vi "eec 6700 Perform Test in Program Mode.vi"() -> ()   [LabVIEW 2014]
doc: "Configures the instrument to Program mode and starts the test.\nThe instrument has 50 memory locations with 9 steps for each memory location.\n\nPress stop button to end the test process.\n\nNote :1. In Firmware version 2.0, the Voltage Limits and Frequency limits are removed from program mode. Its possible to configure the limits in version 1.06 only.\n\n2. Also the Output angle (Start and End) Angle is used as a step parameter in firmware version 2 and system parameter in the firmware version 1.06 respectively.\n\n3. In firmware version 1.06, Enable Surge-Drop Mode is a system parameter (common for all steps and memory. Change in mode affect all steps and memory)\n\n4. In the firmware version 2.0 and above ,surge drop can be used only in the Program Mode and it is a step parameter."
uses:
  <instrlib>/eec 6700/eec 6700.lvlib
panel:
  in  "Timeout (10000 ms)":u32=10000
  in  "Starting Step (1)":i32=1
  in  "Enable Over Current Fold Back (F:Disable)":bool
  in  "Start Angle (0)":i32 min=0 max=359
  in  "End Angle: (0)":i32 min=0 max=359
  in  "Frequency High Limit (500 Hz)":dbl=500.0 min=0.0 max=500.0 format="%.1f"
  in  "Frequency Low Limit (40 Hz)":dbl=40.0 min=0.0 max=500.0 format="%.1f"
  in  "Voltage Low Limit (0 V)":dbl min=0.0 max=400.0 format="%.1f"
  in  "Voltage High Limit (300 V)":dbl=300.0 min=0.0 max=400.0 format="%.1f"
  out "Status Byte Register Cluster":T1={"All Pass"=TRUE, "Fail"=FALSE, "Abort"=FALSE, "Test in Process"=FALSE, "Message Available"=FALSE, "Event Summary Bit"=FALSE, "Not Used"=FALSE, "Prompt"=FALSE}
  in  "Stop":bool
  in  "VISA resource name":refnum<visa-resource-name>="COM1"
  out "Test Meter Data Output":T2={"Memory"=1.0, "Step"=4.0, "Timer (s)"=1.0, "Frequency (Hz)"=60.0, "Voltage (V)"=125.0, "RMS Current (A)"=0.0, "Peak Current (A)"=0.0, "Power (W)"=0.0, "Power Factor"=0.0, "Status"="Pass"} {"Frequency (Hz)" format="%.1f"; "Voltage (V)" format="%.1f"; "RMS Current (A)" format="%.3f"; "Power (W)" format="%.1f"; "Peak Current (A)" format="%.1f"; "Power Factor" format="%.3f"; "Timer (s)" format="%.1f"}
  in  "Memory Cycle (1)":i32=1 min=0 max=9999 step=1
  in  "Memory (1)":i32=1 min=1 max=50 step=1
  in  "Single Step Mode (F:Disable)":bool
  in  "Loop Cycle (1)":i32=1 min=0 max=9999 step=1
  in  "Step Parameters":T3(array[cluster])=[{"Current High Limit (0 A)"=0.0, "Current Peak High Limit (0 A)"=0.0, "Output AC Voltage (115 V) "=115.0, "Enable Step Connection (F:Disable)"=TRUE, "Step (1)"=1, "Step Cycle (1)"=1, "Power Low Limit (0 W)"=0.0, "Power High Limit (0 W)"=0.0, "Power Factor Low Limit (0)"=0.0, "Power Factor High Limit (0)"=0.0, "Current Low Limit (0 A)"=0.0, "Current Peak Low Limit (0 A)"=0.0, "Dwell (1 s)"=3.0, "Ramp Down Time (0 s)"=2.0, "Delay (0.5 s)"=1.0, "Ramp Up Time (0 s)"=2.0, "Surge Drop Duration (0 ms)"=0.0, "Surge Drop Voltage (100 V) "=100.0, "Surge Drop Start Time (0 ms)"=0.0, "Enable  Continuous Surge Drop (F:Disable)"=FALSE, "Output AC Voltage Frequency (60  Hz)"=60.0, "Voltage Range Mode (1:Auto)"=1, "Enable Surge Drop (F:Disable) "=FALSE, "Step Prompt"={"Enable Prompt"=FALSE, "Prompt ( )"=""}}, {"Current High Limit (0 A)"=0.0, "Current Peak High Limit (0 A)"=8.1387e-320, "Output AC Voltage (115 V) "=110.0, "Enable Step Connection (F:Disable)"=TRUE, "Step (1)"=2, "Step Cycle (1)"=1, "Power Low Limit (0 W)"=0.0, "Power High Limit (0 W)"=0.0, "Power Factor Low Limit (0)"=1.35542481148e-312, "Power Factor High Limit (0)"=0.0, "Current Low Limit (0 A)"=0.0, "Current Peak Low Limit (0 A)"=0.0, "Dwell (1 s)"=15.0, "Ramp Down Time (0 s)"=1.0, "Delay (0.5 s)"=0.5, "Ramp Up Time (0 s)"=1.0, "Surge Drop Duration (0 ms)"=0.0, "Surge Drop Voltage (100 V) "=100.0, "Surge Drop Start Time (0 ms)"=0.0, "Enable  Continuous Surge Drop (F:Disable)"=FALSE, "Output AC Voltage Frequency (60  Hz)"=60.0, "Voltage Range Mode (1:Auto)"=1, "Enable Surge Drop (F:Disable) "=FALSE, "Step Prompt"={"Enable Prompt"=FALSE, "Prompt ( )"=""}}, {"Current High Limit (0 A)"=0.0, "Current Peak High Limit (0 A)"=0.0, "Output AC Voltage (115 V) "=120.0, "Enable Step Connection (F:Disable)"=TRUE, "Step (1)"=3, "Step Cycle (1)"=1, "Power Low Limit (0 W)"=0.0, "Power High Limit (0 W)"=0.0, "Power Factor Low Limit (0)"=0.0, "Power Factor High Limit (0)"=0.0, "Current Low Limit (0 A)"=0.0, "Current Peak Low Limit (0 A)"=0.0, "Dwell (1 s)"=1.0, "Ramp Down Time (0 s)"=0.0, "Delay (0.5 s)"=0.5, "Ramp Up Time (0 s)"=0.0, "Surge Drop Duration (0 ms)"=0.0, "Surge Drop Voltage (100 V) "=100.0, "Surge Drop Start Time (0 ms)"=0.0, "Enable  Continuous Surge Drop (F:Disable)"=FALSE, "Output AC Voltage Frequency (60  Hz)"=65.0, "Voltage Range Mode (1:Auto)"=1, "Enable Surge Drop (F:Disable) "=FALSE, "Step Prompt"={"Enable Prompt"=FALSE, "Prompt ( )"=""}}, {"Current High Limit (0 A)"=0.0, "Current Peak High Limit (0 A)"=0.0, "Output AC Voltage (115 V) "=125.0, "Enable Step Connection (F:Disable)"=FALSE, "Step (1)"=4, "Step Cycle (1)"=1, "Power Low Limit (0 W)"=0.0, "Power High Limit (0 W)"=0.0, "Power Factor Low Limit (0)"=0.0, "Power Factor High Limit (0)"=0.0, "Current Low Limit (0 A)"=0.0, "Current Peak Low Limit (0 A)"=0.0, "Dwell (1 s)"=1.0, "Ramp Down Time (0 s)"=0.0, "Delay (0.5 s)"=0.5, "Ramp Up Time (0 s)"=0.0, "Surge Drop Duration (0 ms)"=0.0, "Surge Drop Voltage (100 V) "=100.0, "Surge Drop Start Time (0 ms)"=0.0, "Enable  Continuous Surge Drop (F:Disable)"=FALSE, "Output AC Voltage Frequency (60  Hz)"=60.0, "Voltage Range Mode (1:Auto)"=1, "Enable Surge Drop (F:Disable) "=FALSE, "Step Prompt"={"Enable Prompt"=FALSE, "Prompt ( )"=""}}] {"Voltage Range Mode (1:Auto)" items=["High", "Auto"]; "Output AC Voltage Frequency (60  Hz)" min=45.0 max=500.0 format="%.1p"; "Surge Drop Start Time (0 ms)" min=0.0 max=99.0; "Surge Drop Voltage (100 V)" min=0.0 max=300.0 format="%#.1f"; "Surge Drop Duration (0 ms)" min=0.0 max=99.0; "Ramp Up Time (0 s)" min=0.0 max=999.9 format="%.1f"; "Delay (0.5 s)" min=0.5 max=999.9 format="%.1f"; "Ramp Down Time (0 s)" min=0.0 max=999.9 format="%.1f"; "Dwell (1 s)" min=0.5 max=999.9 format="%.1f"; "Current Peak Low Limit (0 A)" min=0.0 max=152.0 format="%.3f"; "Current Low Limit (0 A)" min=0.0 max=36.8 format="%.3f"; "Power Factor High Limit (0)" min=0.0 max=1.0 format="%.3f"; "Power Factor Low Limit (0)" min=0.0 max=1.0 format="%.3f"; "Power High Limit (0 W)" min=0.0 max=4000.0 format="%.1f"; "Power Low Limit (0 W)" min=0.0 max=4000.0 format="%.1f"; "Step Cycle (1)" min=0 max=9999 step=1; "Step (1)" min=1 max=9 step=1; "Output AC Voltage (115 V)" min=0.0 max=300.0 format="%.1f"; "Current Peak High Limit (0 A)" min=0.0 max=152.0 format="%.3f"; "Current High Limit (0 A)" min=0.0 max=36.8 format="%.3f"}
  out "Error Out":errorcluster
  # "eec 6700 PROGRAM MODE - EXAMPLE"
  # "Note :\n1. Configure the Parameters (Select the instrument VISA resource, voltage etc.,)\n2. Run this VI"
  # "The Step connect mode is used to connect or disconnect one step from another.\nPlease Switch it ON to connect from Step 1 to Step 2."
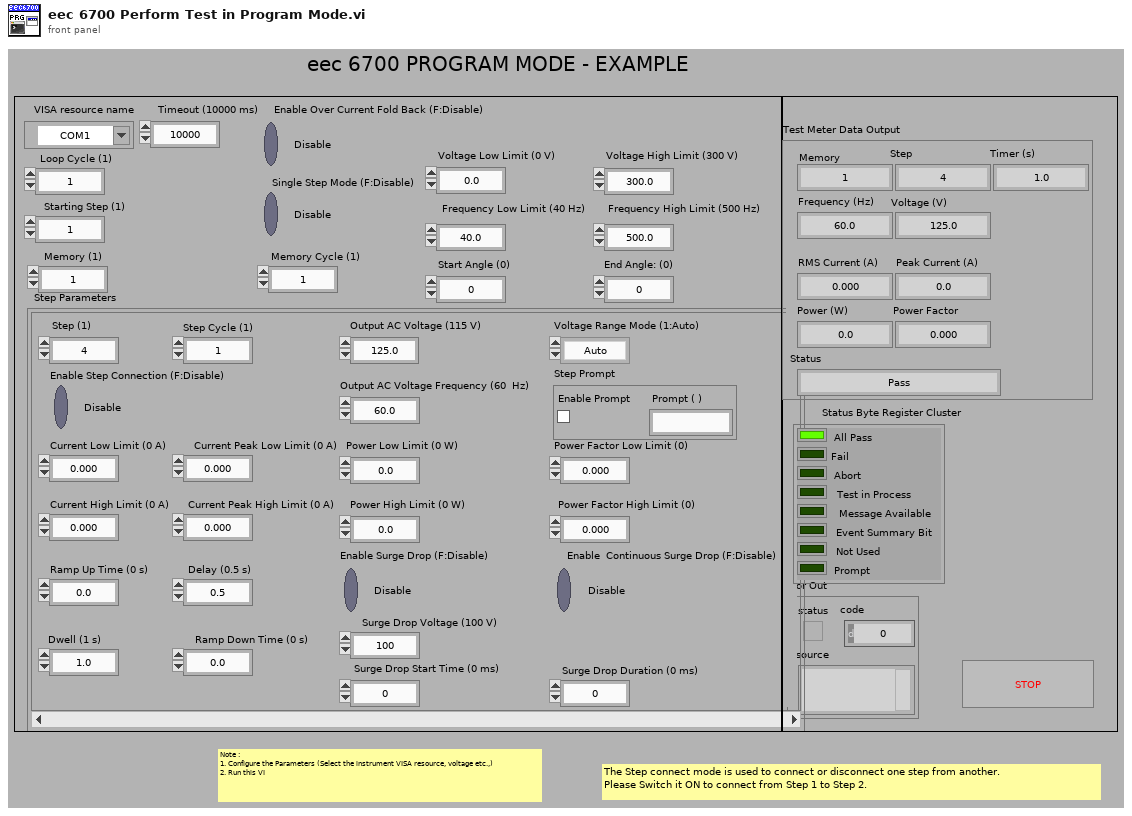
[diagram p1: front panel]
types:
  T1 = cluster{"All Pass":bool, "Fail":bool, "Abort":bool, "Test in Process":bool, "Message Available":bool, "Event Summary Bit":bool, "Not Used":bool, "Prompt":bool}
  T2 = cluster{"Memory":dbl, "Step":dbl, "Timer (s)":dbl, "Frequency (Hz)":dbl, "Voltage (V)":dbl, "RMS Current (A)":dbl, "Peak Current (A)":dbl, "Power (W)":dbl, "Power Factor":dbl, "Status":string}
  T3 = cluster{"Current High Limit (0 A)":dbl, "Current Peak High Limit (0 A)":dbl, "Output AC Voltage (115 V) ":dbl, "Enable Step Connection (F:Disable)":bool, "Step (1)":i32, "Step Cycle (1)":i32, "Power Low Limit (0 W)":dbl, "Power High Limit (0 W)":dbl, "Power Factor Low Limit (0)":dbl, "Power Factor High Limit (0)":dbl, "Current Low Limit (0 A)":dbl, "Current Peak Low Limit (0 A)":dbl, "Dwell (1 s)":dbl, "Ramp Down Time (0 s)":dbl, "Delay (0.5 s)":dbl, "Ramp Up Time (0 s)":dbl, "Surge Drop Duration (0 ms)":dbl, "Surge Drop Voltage (100 V) ":dbl, "Surge Drop Start Time (0 ms)":dbl, "Enable  Continuous Surge Drop (F:Disable)":bool, "Output AC Voltage Frequency (60  Hz)":dbl, "Voltage Range Mode (1:Auto)":u16, "Enable Surge Drop (F:Disable) ":bool, "Step Prompt":cluster{"Enable Prompt":bool, "Prompt ( )":string}}[]
  T4 = cluster{"Baud Rate":u32, "Parity":u16, "Data Bits":u16, "Stop Bits":u16, "Flow Control":u16}
  T5 = cluster{"Enable Prompt":bool, "Prompt ( )":string}
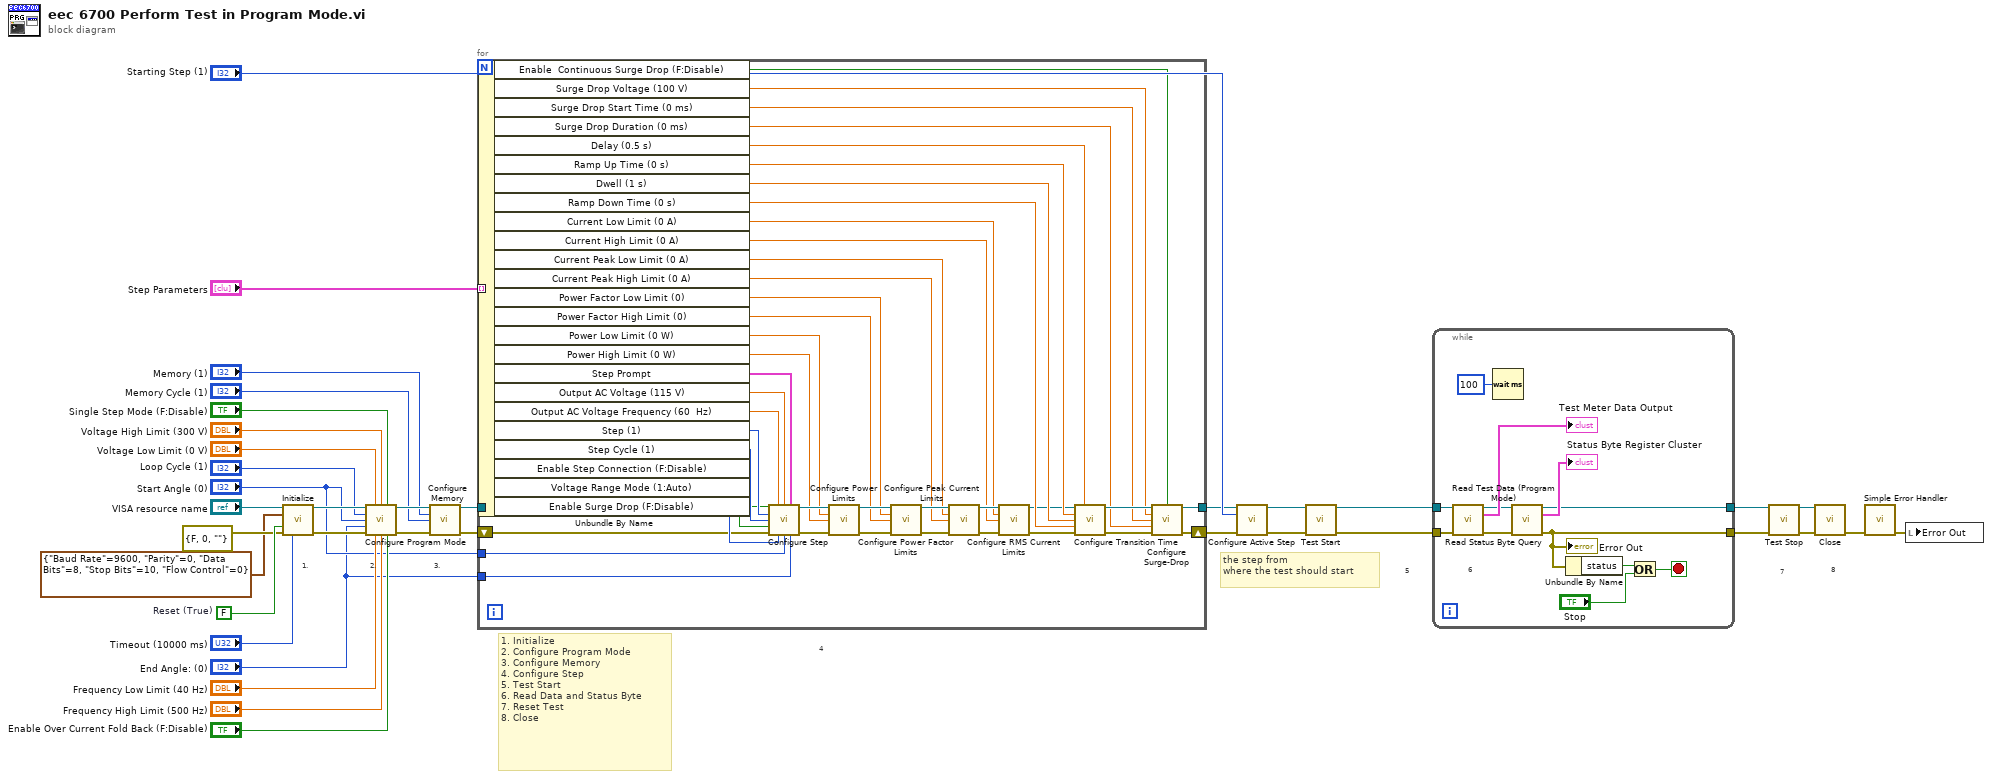
[diagram p0: block diagram]
diagram:
  w34 = FALSE  # Reset (True)
  # "the step from \nwhere the test should start"
  # "5"
  # "4"
  # "1. Initialize\n2. Configure Program Mode\n3. Configure Memory\n4. Configure Step\n5. Test Start\n6. Read Data and Status Byte\n7. Reset Test\n8. Close"
  # "7"
  # "8"
  # "1."
  # "3."
  # "2."
  n1 = call <instrlib>:"Initialize.vi"("VISA resource name"="VISA resource name", "Serial Configuration"=T4 {"Baud Rate"=9600, "Parity"=0, "Data Bits"=8, "Stop Bits"=10, "Flow Control"=0}, "Reset (True)"=w34, "error in (no error)"=errorcluster {"status"=FALSE, "code"=0, "source"=""}, "Timeout (10000 ms)"="Timeout (10000 ms)") -> ("VISA resource name out"=w33:refnum<visa-resource-name>, "error out"=w35:errorcluster)  [unwired: 9 in]
  n2 = call <instrlib>:"Configure Program Mode.vi"("VISA resource name"=w33, "Voltage Low Limit (0 V)"="Voltage Low Limit (0 V)", "Voltage High Limit (300 V)"="Voltage High Limit (300 V)", "Single Step Mode (F:Disable)"="Single Step Mode (F:Disable)", "Loop Cycle (1)"="Loop Cycle (1)", "Start Angle (0)"="Start Angle (0)", "End Angle: (0)"="End Angle: (0)", "error in (no error)"=w35, "Frequency Low Limit (40 Hz)"="Frequency Low Limit (40 Hz)", "Frequency High Limit (500 Hz)"="Frequency High Limit (500 Hz)", "Enable Over Current Fold Back (F:Disable)"="Enable Over Current Fold Back (F:Disable)") -> ("VISA resource name out"=w32:refnum<visa-resource-name>, "error out"=w31:errorcluster)  [unwired: 3 in]
  n3 = call <instrlib>:"Configure Memory.vi"("VISA resource name"=w32, "Memory (1)"="Memory (1)", "Memory Cycle (1)"="Memory Cycle (1)", "error in (no error)"=w31) -> ("VISA resource name out"=w8:refnum<visa-resource-name>, "error out"=w7:errorcluster)  [unwired: 10 in]
  n4 = for {
    tunnel: "Step Parameters" -> [w77] mode=indexing
    shift-right: [w79] -> w3
    shift-left: w7 -> [w41]
    tunnel: [w78] -> w4
    tunnel: w8 -> [w42]
    tunnel: "Start Angle (0)" -> [w40]
    tunnel: "End Angle: (0)" -> [w39]
    n5 = Unbundle By Name(w77) -> ("Enable  Continuous Surge Drop (F:Disable)"=w45:bool, "Surge Drop Voltage (100 V)"=w53:dbl, "Surge Drop Start Time (0 ms)"=w54:dbl, "Surge Drop Duration (0 ms)"=w55:dbl, "Delay (0.5 s)"=w65:dbl, "Ramp Up Time (0 s)"=w64:dbl, "Dwell (1 s)"=w59:dbl, "Ramp Down Time (0 s)"=w58:dbl, "Current Low Limit (0 A)"=w46:dbl, "Current High Limit (0 A)"=w37:dbl, "Current Peak Low Limit (0 A)"=w52:dbl, "Current Peak High Limit (0 A)"=w51:dbl, "Power Factor Low Limit (0)"=w72:dbl, "Power Factor High Limit (0)"=w71:dbl, "Power Low Limit (0 W)"=w70:dbl, "Power High Limit (0 W)"=w69:dbl, "Step Prompt"=w38:T5, "Output AC Voltage (115 V)"=w56:dbl, "Output AC Voltage Frequency (60  Hz)"=w57:dbl, "Step (1)"=w44:i32, "Step Cycle (1)"=w67:i32, "Enable Step Connection (F:Disable)"=w68:bool, "Voltage Range Mode (1:Auto)"=w66:u16, "Enable Surge Drop (F:Disable)"=w43:bool)
    n6 = call <instrlib>:"Configure Step.vi"("VISA resource name"=w42, "Output AC Voltage Frequency (60  Hz)"=w57, "Output AC Voltage (115 V)"=w56, "Step Prompt"=w38, "Step (1)"=w44, "Step Cycle (1)"=w67, "Enable Step Connection (F:Disable)"=w68, "error in (no error)"=w41, "Voltage Range Mode (1:Auto)"=w66, "Start Angle (0)"=w40, "End Angle: (0)"=w39) -> ("VISA resource name out"=w76:refnum<visa-resource-name>, "error out"=w75:errorcluster)  [unwired: 3 in]
    n7 = call <instrlib>:"Configure Power Limits.vi"("VISA resource name"=w76, "Power Low Limit (0 W)"=w70, "Power High Limit (0 W)"=w69, "error in (no error)"=w75) -> ("VISA resource name out"=w74:refnum<visa-resource-name>, "error out"=w73:errorcluster)  [unwired: 10 in]
    n8 = call <instrlib>:"Configure Power Factor Limits.vi"("VISA resource name"=w74, "Power Factor Low Limit (0)"=w72, "Power Factor High Limit (0)"=w71, "error in (no error)"=w73) -> ("VISA resource name out"=w63:refnum<visa-resource-name>, "error out"=w62:errorcluster)  [unwired: 10 in]
    n9 = call <instrlib>:"Configure Peak Current Limits.vi"("VISA resource name"=w63, "Current Peak Low Limit (0 A)"=w52, "Current Peak High Limit (0 A)"=w51, "error in (no error)"=w62) -> ("VISA resource name out"=w50:refnum<visa-resource-name>, "error out"=w49:errorcluster)  [unwired: 10 in]
    n10 = call <instrlib>:"Configure RMS Current Limits.vi"("VISA resource name"=w50, "Current Low Limit (0 A)"=w46, "Current High Limit (0 A)"=w37, "error in (no error)"=w49) -> ("VISA resource name out"=w47:refnum<visa-resource-name>, "error out"=w48:errorcluster)  [unwired: 10 in]
    n11 = call <instrlib>:"Configure Transition Time.vi"("VISA resource name"=w47, "Delay (0.5 s)"=w65, "Ramp Up Time (0 s)"=w64, "Dwell (1 s)"=w59, "Ramp Down Time (0 s)"=w58, "error in (no error)"=w48) -> ("VISA resource name out"=w60:refnum<visa-resource-name>, "error out"=w61:errorcluster)  [unwired: 8 in]
    n12 = call <instrlib>:"Configure Surge-Drop.vi"("VISA resource name"=w60, "Enable Surge Drop (F:Disable)"=w43, "Enable  Continuous Surge Drop (F:Disable)"=w45, "Surge Drop Voltage (100 V)"=w53, "Surge Drop Start Time (0 ms)"=w54, "Surge Drop Duration (0 ms)"=w55, "error in (no error)"=w61) -> ("VISA resource name out"=w78:refnum<visa-resource-name>, "error out"=w79:errorcluster)  [unwired: 7 in]
  }
  n13 = call <instrlib>:"Configure Active Step.vi"("VISA resource name"=w4, "Step (1)"="Starting Step (1)", "error in (no error)"=w3) -> ("VISA resource name out"=w16:refnum<visa-resource-name>, "error out"=w15:errorcluster)  [unwired: 11 in]
  n14 = call <instrlib>:"Test Start.vi"("VISA resource name"=w16, "error in (no error)"=w15) -> ("VISA resource name out"=w2:refnum<visa-resource-name>, "error out"=w1:errorcluster)  [unwired: 12 in]
  n15 = while {
    tunnel: [w84] -> w24
    tunnel: [w80] -> w22
    tunnel: w2 -> [w91]
    tunnel: w1 -> [w90]
    stop <- w81 stop-if-true
    # "6"
    n16 = call <instrlib>:"Read Test Data (Program Mode).vi"("VISA resource name"=w91, "error in (no error)"=w90) -> ("VISA resource name out"=w85:refnum<visa-resource-name>, "Test Meter Data Output"=→"Test Meter Data Output":T2, "error out"=w86:errorcluster)  [unwired: 11 in]
    n17 = Wait (ms)(milliseconds to wait=u32 100) -> ()  [unwired: 1 out]
    n18 = call <instrlib>:"Read Status Byte Query.vi"("VISA resource name"=w85, "error in (no error)"=w86) -> ("VISA resource name out"=w84:refnum<visa-resource-name>, "Status Byte Register"=→"Status Byte Register Cluster":T1, "error out"=w80:errorcluster)  [unwired: 11 in]
    "Error Out" <- w80
    n19 = Unbundle By Name(w80) -> ("status"=w83:bool)
    n20 = Or(x=w83, y="Stop") -> (x .or. y?=w81:bool)
  }
  n21 = call <instrlib>:"Test Stop.vi"("VISA resource name"=w24, "error in (no error)"=w22) -> ("VISA resource name out"=w25:refnum<visa-resource-name>, "error out"=w23:errorcluster)  [unwired: 12 in]
  n22 = call <instrlib>:"Close.vi"("VISA resource name"=w25, "error in (no error)"=w23) -> ("error out"=w36:errorcluster)  [unwired: 13 in]
  n23 = call <vilib>:"Simple Error Handler.vi"("error in (no error)"=w36) -> ("error out"=w6:errorcluster)  [unwired: 4 in, 4 out]
  n24 = local write "Error Out"(w6) -> ()
